vi "PRL BUFFER Cut from Complex 2D Array.vi"(9 "Cut Index":i32, 10 "Signal Index":i32, 11 "Array In":csg[][](array[numeric])) -> (3 "Array Out":csg[](array[numeric]))   [LabVIEW 2013, in "PMU Recorder Light.lvlib"]
uses:
  PMU Recorder Light.lvlib
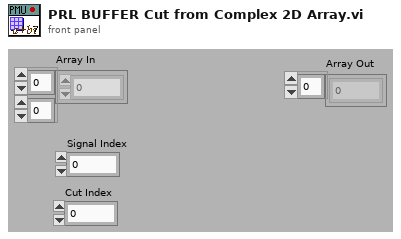
[diagram p1: front panel]
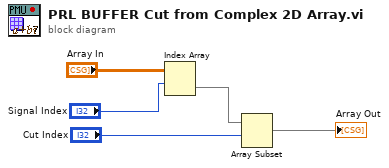
[diagram p0: block diagram]
diagram:
  n1 = Index Array(array="Array In", index (row)="Signal Index") -> (element=w3:csg[])  [unwired: 1 in]
  n2 = Array Subset(array=w3, index="Cut Index") -> (→"Array Out":csg[])  [unwired: 1 in]
